vi "Account FGV Unit Testing.vi"() -> ()   [LabVIEW 2012]
uses:
  Account FGV/Account Methods.ctl
panel:
  out "Account Balance":dbl
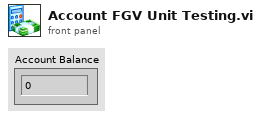
[diagram p1: front panel]
types:
  T1 = typedef "Account Methods.ctl" = enum16{"Deposit", "Withdraw", "Get Balance", "Clear Balance"}
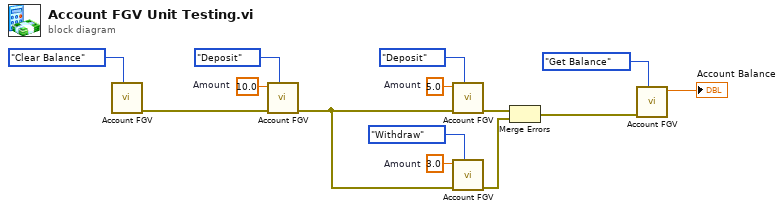
[diagram p0: block diagram]
diagram:
  w7 = 3.0  # Amount
  w10 = 5.0  # Amount
  w11 = 10.0  # Amount
  n1 = call "Account FGV.vi"("Account Methods"=Account_Methods."Clear Balance" ("Bank Commands")) -> ("error out"=w12:errorcluster)  [unwired: 2 in, 8 out]
  n2 = call "Account FGV.vi"("Account Methods"=Account_Methods."Deposit" ("Bank Commands"), "error in"=w12, "Amount"=w11) -> ("error out"=w4:errorcluster)  [unwired: 8 out]
  n3 = call "Account FGV.vi"("Account Methods"=Account_Methods."Deposit" ("Bank Commands"), "error in"=w4, "Amount"=w10) -> ("error out"=w3:errorcluster)  [unwired: 8 out]
  n4 = call "Account FGV.vi"("Account Methods"=Account_Methods."Withdraw" ("Bank Commands"), "error in"=w4, "Amount"=w7) -> ("error out"=w2:errorcluster)  [unwired: 8 out]
  n5 = Merge Errors(w3, w2) -> (w1:errorcluster)
  n6 = call "Account FGV.vi"("Account Methods"=Account_Methods."Get Balance" ("Bank Commands"), "error in"=w1) -> ("Account Balance"=→"Account Balance":dbl)  [unwired: 1 in, 8 out]
